vi "UpdateSysResourcesToMap.vi"(8 "error in (no error)":errorcluster, 11 "map in":T4) -> (0 "error out":errorcluster, 2 "system resources":T1 {"CPU Loads"."ISR (%)" format="%#.2f"; "CPU Loads"."Idle (%)" format="%#.2f"; "CPU Loads"."Background (%)" format="%#.2f"; "CPU Loads"."Normal (%)" format="%#.2f"; "CPU Loads"."Above Normal (%)" format="%#.2f"; "CPU Loads"."High (%)" format="%#.2g"; "CPU Loads"."Timed Structures (%)" format="%#.2g"; "CPU Loads"."Time Critical (%)" format="%#.2g"; "CPU Loads"."Total (%)" format="%#.2g"}, 3 "map out":T4)   [LabVIEW 2017, in "SystemInfoProcess.lvlib"]
uses:
  <vilib>/addons/SystemInfoProcess/SystemInfoProcess.lvlib
  <vilib>/addons/PointValueMap/controls/PointMap.ctl
  <vilib>/addons/SystemInfoProcess/controls/SystemResources.ctl
  <vilib>/addons/SystemInfoProcess/controls/Utilization.ctl
  <vilib>/addons/SystemInfoProcess/controls/CPULoad.ctl
  <vilib>/addons/PointValueMap/subVIs/Point_Write_variant.vi
  <resource>/objmgr/nisysapi.rc
  <vilib>/addons/PointValueMap/PointValueMap.lvlib
  <vilib>/Analysis/NI_AALBase.lvlib
  <vilib>/Analysis/baseanly.llb/Mean (DBL).vi
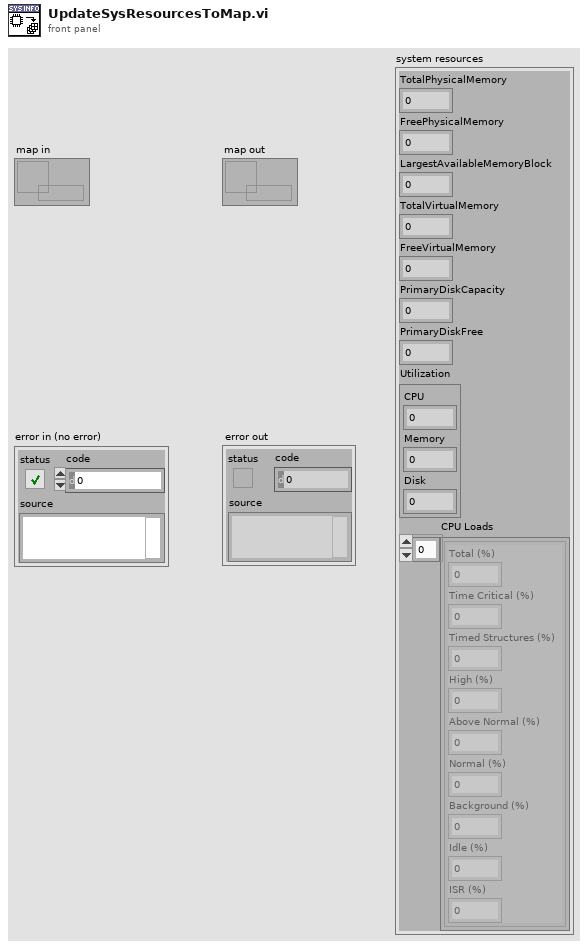
[diagram p1: front panel]
types:
  T1 = typedef "SystemInfoProcess.lvlib/SystemResources.ctl" = cluster{"TotalPhysicalMemory":dbl, "FreePhysicalMemory":dbl, "LargestAvailableMemoryBlock":dbl, "TotalVirtualMemory":dbl, "FreeVirtualMemory":dbl, "PrimaryDiskCapacity":dbl, "PrimaryDiskFree":dbl, "Utilization":T2, "CPU Loads":T3[]}
  T2 = typedef "SystemInfoProcess.lvlib/Utilization.ctl" = cluster{"CPU":dbl, "Memory":dbl, "Disk":dbl}
  T3 = typedef "SystemInfoProcess.lvlib/CPULoad.ctl" = cluster{"Total (%)":dbl, "Time Critical (%)":dbl, "Timed Structures (%)":dbl, "High (%)":dbl, "Above Normal (%)":dbl, "Normal (%)":dbl, "Background (%)":dbl, "Idle (%)":dbl, "ISR (%)":dbl}
  T4 = typedef "PointValueMap.lvlib/PointMap.ctl" = refnum<data-value>
  T5 = typedef "NI_Real-Time Target Support.lvlib/RT CPU Load.ctl" = cluster{"Total (%)":dbl, "Time Critical (%)":dbl, "Timed Structures (%)":dbl, "High (%)":dbl, "Above Normal (%)":dbl, "Normal (%)":dbl, "Background (%)":dbl, "Idle (%)":dbl, "ISR (%)":dbl}
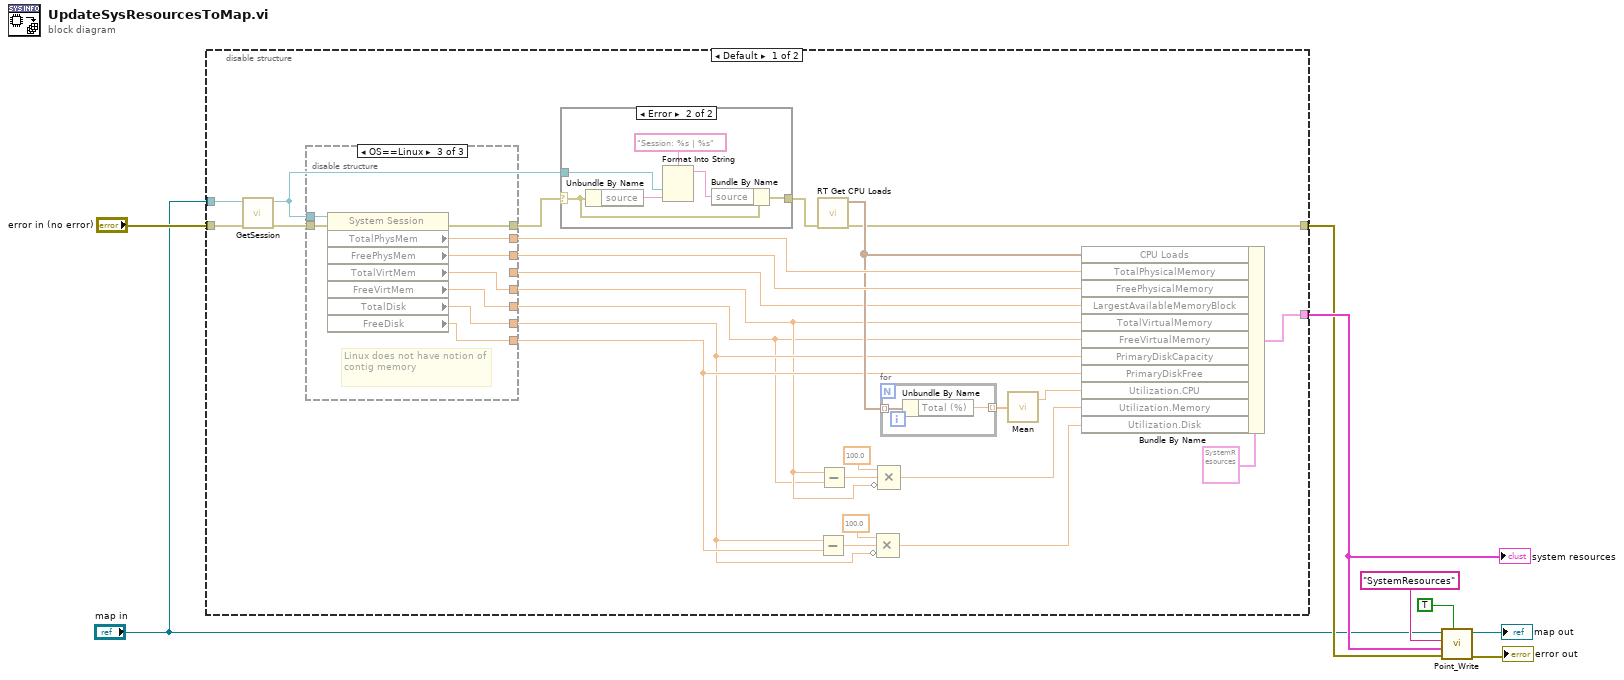
[diagram p0: block diagram]
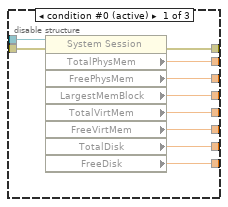
[diagram p3: hidden frame]
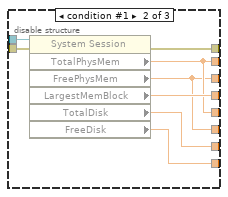
[diagram p4: hidden frame]
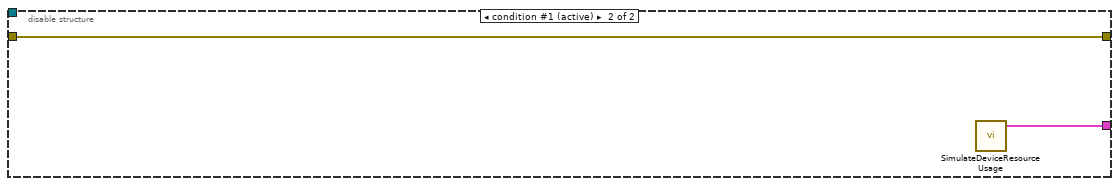
[diagram p5: hidden frame]
diagram:
  n1 = disable-structure shown="Default" {
    disable-tunnel: "error in (no error)" -> [w18 w71]
    disable-tunnel: [w32 w70] -> w4
    disable-tunnel: [w12 w71] -> w3
    disable-tunnel: "map in" -> [w16 _]
    frame condition #0 {
      n2 = call <vilib>:"GetSession.vi"("error in (no error)"=w18, "map"=w16) -> ("error out"=w17:errorcluster, "session"=w9:refnum<k21>)  [unwired: 8 in]
      n3 = disable-structure shown="OS==Linux" {
        disable-tunnel: w9 -> [w50 w58 w67]
        disable-tunnel: w17 -> [w49 w57 w66]
        disable-tunnel: [w48 w56 w65] -> w11
        disable-tunnel: [w47 w55 _] -> w15
        disable-tunnel: [w46 w52 w64] -> w14
        disable-tunnel: [w45 w51 w63] -> w13
        disable-tunnel: [w44 w51 w62] -> w29
        disable-tunnel: [w43 w52 w61] -> w28
        disable-tunnel: [w42 w54 w60] -> w21
        disable-tunnel: [w41 w53 w59] -> w20
        frame condition #0 (active) {
          n4 = property class="System Session"(reference=w50, error in=w49) -> (error out=w48:errorcluster, "TotalPhysMem"=w43:dbl, "FreePhysMem"=w44:dbl, "LargestMemBlock"=w47:dbl, "TotalVirtMem"=w46:dbl, "FreeVirtMem"=w45:dbl, "TotalDisk"=w41:dbl, "FreeDisk"=w42:dbl)  [unwired: 1 out]
        }
        frame condition #1 {
          n5 = property class="System Session"(reference=w58, error in=w57) -> (error out=w56:errorcluster, "TotalPhysMem"=w52:dbl, "FreePhysMem"=w51:dbl, "LargestMemBlock"=w55:dbl, "TotalDisk"=w53:dbl, "FreeDisk"=w54:dbl)  [unwired: 1 out]
        }
        frame condition #2 {
          # "Linux does not have notion of contig memory"
          n6 = property class="System Session"(reference=w67, error in=w66) -> (error out=w65:errorcluster, "TotalPhysMem"=w61:dbl, "FreePhysMem"=w62:dbl, "TotalVirtMem"=w64:dbl, "FreeVirtMem"=w63:dbl, "TotalDisk"=w59:dbl, "FreeDisk"=w60:dbl)  [unwired: 1 out]
        }
      }
      n7 = case shown="Error" w11 {
        selector: w11 -> [w34 w37]
        tunnel: [w34 w35] -> w10
        tunnel: w9 -> [_ w38]
        frame No Error {
        }
        frame Error {
          n8 = Unbundle By Name(w37) -> ("source"=w39:string)
          n9 = Format Into String(format string="Session: %s | %s", w38, w39) -> (resulting string=w36:string)  [unwired: 2 in, 1 out]
          n10 = Bundle By Name(cluster=w37, "source"=w36) -> (w35:errorcluster)
        }
      }
      n11 = call <vilib>:"RT Get CPU Loads.vi"("error in (no error)"=w10) -> ("error out"=w12:errorcluster, "CPU loads"=w26:T5[])  [unwired: 9 in]
      n12 = Subtract(x=w20, y=w21) -> (x-y=w23:dbl)
      n13 = Subtract(x=w14, y=w13) -> (x-y=w30:dbl)
      n14 = Compound Arithmetic op=MULTIPLY(100.0 ("y"), w23, invert w20) -> (w19:dbl)
      n15 = Compound Arithmetic op=MULTIPLY(100.0 ("y"), w30, invert w14) -> (w27:dbl)
      n16 = for {
        tunnel: w26 -> [w69] mode=indexing
        tunnel: [w68] -> w25 mode=indexing
        n17 = Unbundle By Name(w69) -> ("Total (%)"=w68:dbl)
      }
      n18 = call-poly <vilib>:"Mean.vi"("X"=w25) -> ("mean"=w24:dbl)  [unwired: 1 out]
      n19 = Bundle By Name(cluster=T1 {"TotalPhysicalMemory"=0.0, "FreePhysicalMemory"=0.0, "LargestAvailableMemoryBlock"=0.0, "TotalVirtualMemory"=0.0, "FreeVirtualMemory"=0.0, "PrimaryDiskCapacity"=0.0, "PrimaryDiskFree"=0.0, "Utilization"={"CPU"=0.0, "Memory"=0.0, "Disk"=0.0}, "CPU Loads"=[]} ("system resources"), "CPU Loads"=w26, "TotalPhysicalMemory"=w28, "FreePhysicalMemory"=w29, "LargestAvailableMemoryBlock"=w15, "TotalVirtualMemory"=w14, "FreeVirtualMemory"=w13, "PrimaryDiskCapacity"=w20, "PrimaryDiskFree"=w21, "Utilization.CPU"=w24, "Utilization.Memory"=w27, "Utilization.Disk"=w19) -> (w32:T1)
    }
    frame condition #1 (active) {
      n20 = call <vilib>:"SimulateDeviceResourceUsage.vi"() -> ("system resources"=w70:T1)  [unwired: 11 in]
    }
  }
  "system resources" <- w4
  n21 = call-poly <vilib>:"Point_Write.vi"("Auto Create?"=TRUE, "Error In"=w3, "Value"=w4, "Tag"="SystemResources", "Map"="map in") -> ("Error Out"=→"error out":errorcluster, "Map Out"=→"map out":T4)  [unwired: 5 in]
